vi "Draw_Text.vi"(7 "Text Settings":cluster{"Font":T1, "Alignment":T2, "Size":T3} {"Alignment" items=["left", "center", "right"]}, 8 "Text Color":T4, 10 "Upper Limit":T6, 11 "Text":string) -> (2 "Text Rect Out":T5, 3 "Empty Picture Out":picture)   [LabVIEW 2021]
uses:
  <vilib>/Utility/miscctls.llb/LVPoint32TypeDef.ctl
  vi.lib/LabVIEW Icon API/lv_icon/Controls/IEColor.ctl
  vi.lib/LabVIEW Icon API/lv_icon/Controls/Font.ctl
  vi.lib/LabVIEW Icon API/lv_icon/Controls/Alignment.ctl
  TypeDefs/Num_Font Size.ctl
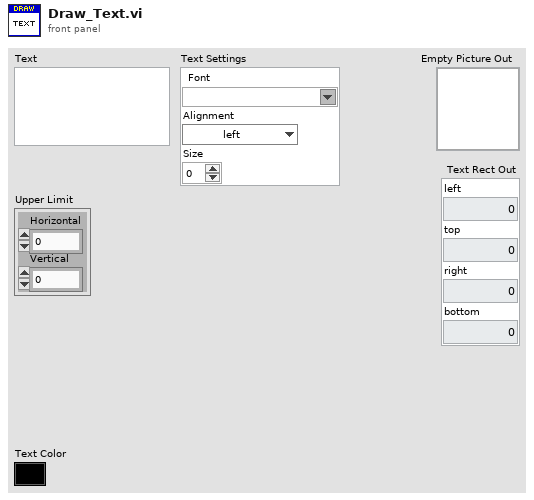
[diagram p1: front panel]
types:
  T1 = typedef "Font.ctl" = string
  T2 = typedef "Alignment.ctl" = u16
  T3 = typedef "Num_Font Size.ctl" = u8
  T4 = typedef "IEColor.ctl" = u32
  T5 = cluster{"left":i16, "top":i16, "right":i16, "bottom":i16}
  T6 = typedef "LVPoint32TypeDef.ctl" = cluster{"Horizontal":i32, "Vertical":i32}
  T7 = enum16{"User-specified Font", "Application Font", "System Font", "Dialog Font"}
  T8 = cluster{"Font Name:":string, "Size":i16, "Strikeout?":bool, "Italic?":bool, "Underline?":bool, "Outline?":bool, "Shadow?":bool, "Bold?":bool}
  T9 = cluster{"horizontal":enum16{"left", "center", "right"}, "vertical":enum16{"top", "center", "bottom"}}
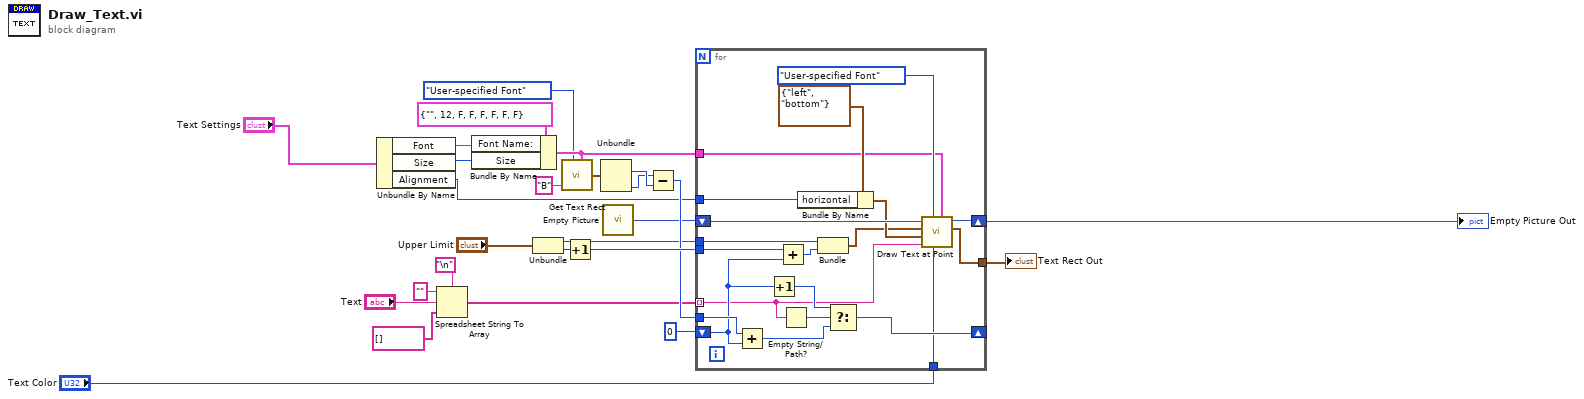
[diagram p0: block diagram]
diagram:
  n1 = Unbundle By Name("Text Settings") -> ("Font"=w9:T1, "Size"=w8:T3, "Alignment"=w12:T2)
  n2 = Spreadsheet String To Array(delimiter (Tab)="\n", format string="", spreadsheet string="Text", array type (2D Dbl)=string[] []) -> (array=w3:string[])
  n3 = Bundle By Name(cluster=T8 {"Font Name:"="", "Size"=12, "Strikeout?"=FALSE, "Italic?"=FALSE, "Underline?"=FALSE, "Outline?"=FALSE, "Shadow?"=FALSE, "Bold?"=FALSE} ("[user-specified font]"), "Font Name:"=w9, "Size"=w8) -> (w18:T8)
  n4 = Unbundle("Upper Limit") -> ("Horizontal"=w5:i32, "Vertical"=w6:i32)
  n5 = call <vilib>:"Get Text Rect.vi"("desired font(Application)"=T7."User-specified Font", "text"="B", "[user-specified font]"=w18) -> ("rect"=w14:T5)  [unwired: 3 in, 3 out]
  n6 = Increment(x=w6) -> (x+1=w21:i32)
  n7 = Unbundle(w14) -> ("top"=w17:i16, "bottom"=w16:i16)  [unwired: 2 out]
  n8 = call "Empty Picture"() -> ("empty picture"=w4:picture)
  n9 = Subtract(x=w16, y=w17) -> (x-y=w19:i16)
  n10 = for {
    tunnel: w3 -> [w29] mode=indexing
    shift-right: [w45] -> w25
    shift-left: w4 -> [w46]
    tunnel: w5 -> [w41]
    tunnel: w21 -> [w39]
    tunnel: w12 -> [w37]
    tunnel: w18 -> [w36]
    shift-right: [w31] -> _
    shift-left: 0 -> [w33]
    tunnel: w19 -> [w34]
    tunnel: [w28] -> w23
    tunnel: "Text Color" -> [w27]
    n11 = Add(x=w34, y=w33) -> (x+y=w32:i32)
    n12 = Increment(x=w33) -> (x+1=w35:i32)
    n13 = Add(x=w39, y=w33) -> (x+y=w40:i32)
    n14 = Empty String/Path?(string/path=w29) -> (empty?=w30:bool)
    n15 = Bundle By Name(cluster=T9 {"horizontal"=enum."left", "vertical"=enum."bottom"} ("alignment(left, top)"), "horizontal"=w37) -> (w43:T9)
    n16 = Bundle("Horizontal"=w41, w40) -> (w38:cluster{"Horizontal":i32, i32})  [unwired: 1 out]
    n17 = Select(t=w35, s=w30, f=w32) -> (s? t:f=w31:i32)
    n18 = call <vilib>:"Draw Text at Point.vi"("[user-specified font]"=w36, "text color(black)"=w27, "desired font(Application)"=T7."User-specified Font", "text"=w29, "alignment(left, top)"=w43, "origin"=w38, "picture"=w46) -> ("text rect"=w28:T5, "new picture"=w45:picture)  [unwired: 2 in, 1 out]
  }
  "Empty Picture Out" <- w25
  "Text Rect Out" <- w23
